vi "Event-driven Scenario (Event Method).vi"() -> ()   [LabVIEW 2012]
panel:
  out "Waveform Graph":dynamicdata(graph)
  in  "Acquire Data":bool
  out "Temperature (deg F)":dbl=32.0
  in  "Temperature (deg C)":dbl
  in  "Time Check":bool
  out "current time":timestamp
  in  "Stop":bool
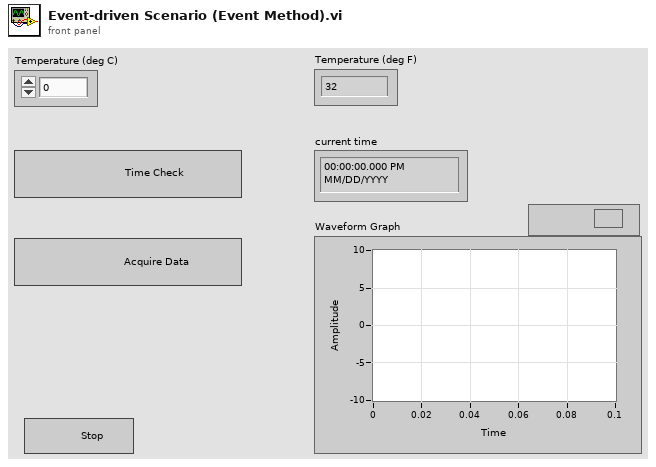
[diagram p1: front panel]
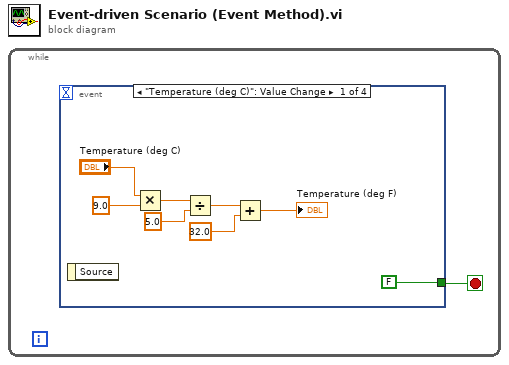
[diagram p0: block diagram]
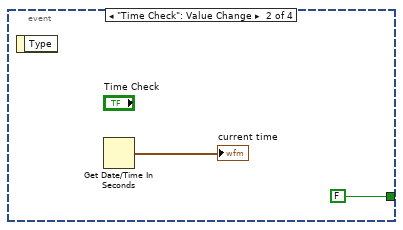
[diagram p2: hidden frame]
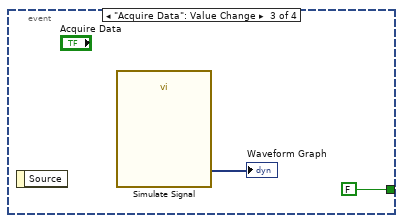
[diagram p3: hidden frame]
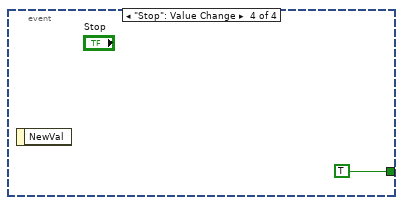
[diagram p4: hidden frame]
diagram:
  n1 = while {
    stop <- w1 stop-if-true
    n2 = event shown="[0] \"Temperature (deg C)\": Value Change" {
      selector: _ -> [_ _ _ _]
      dyn-events: _ -> [_ _ _ _]
      timeout: _ -> [_ _ _ _]
      tunnel: [FALSE FALSE FALSE TRUE] -> w1
      event "Temperature (deg C)": Value Change {
        n3 = event-data() -> ()  [unwired: 1 in, 1 out]
        n4 = Multiply(x="Temperature (deg C)", y=9.0) -> (x*y=w7:dbl)
        n5 = Divide(x=w7, y=5.0) -> (x/y=w5:dbl)
        n6 = Add(x=w5, y=32.0) -> (x+y=→"Temperature (deg F)":dbl)
      }
      event "Time Check": Value Change {
        n7 = event-data() -> ()  [unwired: 1 in, 1 out]
        n8 = Get Date/Time In Seconds() -> (seconds since 1Jan1904=→"current time":timestamp)
      }
      event "Acquire Data": Value Change {
        n9 = event-data() -> ()  [unwired: 1 in, 1 out]
        n10 = call "Simulate Signal"() -> ("Sine with Uniform Noise"=→"Waveform Graph":dynamicdata)  [unwired: 14 in, 1 out]
      }
      event "Stop": Value Change {
        n11 = event-data() -> ()  [unwired: 1 in, 1 out]
      }
    }
  }
